vi "AMB_Global.gbl.vi"() -> ()   [LabVIEW 2017]
doc: "This is used to keep track of the CAN setup (TCP/IP tunneling or direct CAN) and contains the ABM# and Bus# when TCP/IP communication is used."
panel:
  out "Bus#":u16
  out "ABM#":i16
  in  "TCP":bool
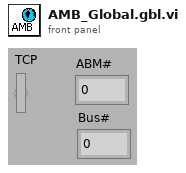
[diagram p1: front panel]
diagram:
